vi "Destroy.vi"(8 "error in (no error)":errorcluster, 11 "CIFPlugin in":refnum<class "Template_Plugin.lvclass">) -> (0 "error out":errorcluster, 3 "CIFPlugin out":refnum<class "Template_Plugin.lvclass">)   [LabVIEW 2021, in "Template_Plugin.lvclass"]
uses:
  Template_Plugin.lvclass
  Template_Plugin.lvclass/Template_Plugin.ctl
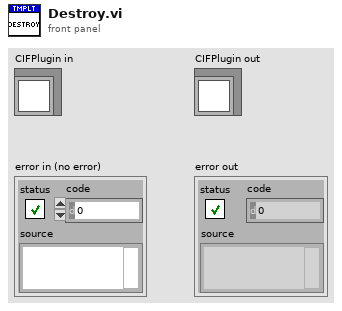
[diagram p1: front panel]
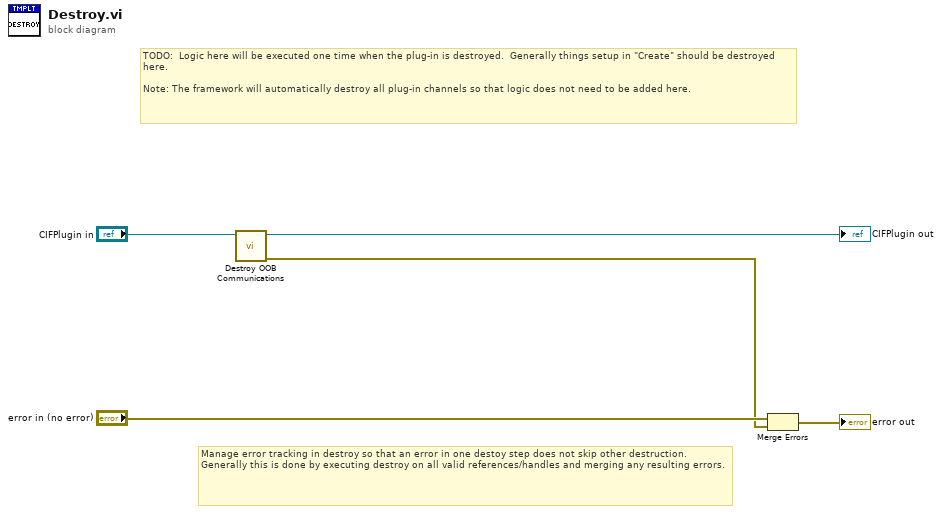
[diagram p0: block diagram]
diagram:
  # "TODO:  Logic here will be executed one time when the plug-in is destroyed.  Generally things setup in \"Create\" should be destroyed here.  \n\nNote: The framework will automatically destroy all plug-in channels so that logic does not need to be added here."
  # "Manage error tracking in destroy so that an error in one destoy step does not skip other destruction.   Generally this is done by executing destroy on all valid references/handles and merging any resulting errors."
  n1 = call "Destroy OOB Communications.vi"("CIFPlugin in"="CIFPlugin in") -> ("error out"=w1:errorcluster, "CIFPlugin out"=→"CIFPlugin out":refnum<class "Template_Plugin.lvclass">)  [unwired: 9 in]
  n2 = Merge Errors("error in (no error)", w1) -> (→"error out":errorcluster)
